vi "Gather_Files_containing.vi"() -> ()   [LabVIEW 2010]
panel:
  in  "Does Contain":bool
  in  "Copy to folder":path
  in  "Names containing":string
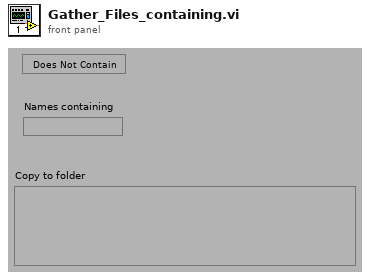
[diagram p1: front panel]
types:
  T1 = enum32{"existing file", "new file", "new or existing file", "existing dir", "new dir", "new or existing dir", "existing file (use LLBs)", "new file (use LLBs)", "new or existing file (use LLBs)", "new or existing file or directory (use LLBs)"}
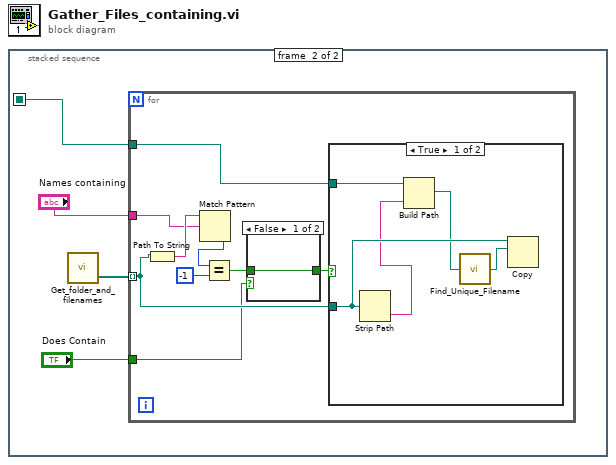
[diagram p0: block diagram]
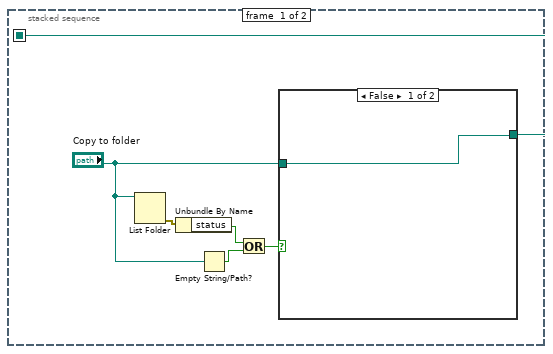
[diagram p2: hidden frame]
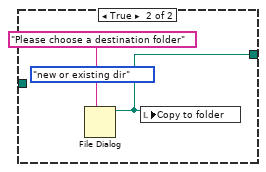
[diagram p3: hidden frame]
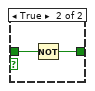
[diagram p4: hidden frame]
diagram:
  n1 = stacked-sequence {
    seq-local: [w5 _] -> [_ w11]
    frame #0 {
      n2 = List Folder(path="Copy to folder") -> (error out=w6:errorcluster)  [unwired: 3 in, 3 out]
      n3 = Unbundle By Name(w6) -> ("status"=w2:bool)
      n4 = Empty String/Path?(string/path="Copy to folder") -> (empty?=w3:bool)
      n5 = Or(x=w2, y=w3) -> (x .or. y?=w1:bool)
      n6 = case shown="False" w1 {
        tunnel: [w7 w9] -> w5
        tunnel: "Copy to folder" -> [w7 _]
        frame False {
        }
        frame True {
          (unwired) T1."new or existing dir" ("select mode (2)")
          n7 = File Dialog(7:"Please choose a destination folder" ("prompt")) -> (3:w9:path)  [unwired: 6 in, 3 out]
          n8 = local write "Copy to folder"(w9) -> ()
        }
      }
    }
    frame #1 {
      n9 = call "Get_folder_and_filenames.vi"() -> ("Files"=w13:path[])  [unwired: 1 in, 1 out]
      n10 = for {
        tunnel: w13 -> [w20] mode=indexing
        tunnel: "Names containing" -> [w21]
        tunnel: w11 -> [w19]
        tunnel: "Does Contain" -> [w16]
        n11 = Path To String(path=w20) -> (string=w22:string)
        n12 = Match Pattern(string=w22, regular expression=w21) -> (offset past match=w18:i32)  [unwired: 1 in, 3 out]
        n13 = Equal?(x=w18, y=-1) -> (x = y?=w14:bool)
        n14 = case shown="False" w16 {
          tunnel: [w23 w24] -> w15
          tunnel: w14 -> [w23 w25]
          frame False {
          }
          frame True {
            n15 = Not(x=w25) -> (.not. x?=w24:bool)
          }
        }
        n16 = case shown="True" w15 {
          tunnel: w20 -> [w30 _]
          tunnel: w19 -> [w29 _]
          frame True {
            n17 = Strip Path(path=w30) -> (name=w28:string)  [unwired: 1 out]
            n18 = Build Path(base path=w29, name or relative path=w28) -> (appended path=w27:path)
            n19 = call "Find_Unique_Filename.vi"("Path In"=w27) -> ("Unique Path Out"=w26:path)  [unwired: 2 in]
            n20 = Copy(10:w26, 11:w30) -> ()  [unwired: 3 in, 3 out]
          }
          frame False {
          }
        }
      }
    }
  }
